vi "Platform Plugin Folder.vi"() -> (2 "Path":path)   [LabVIEW 2020, in "PicoG-Core.lvlib" / "PlatformManager.lvclass"]
uses:
  PlatformManager.lvclass
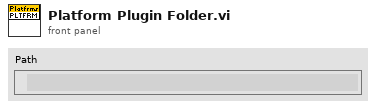
[diagram p1: front panel]
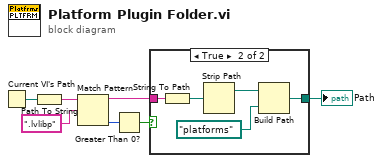
[diagram p0: block diagram]
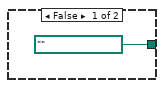
[diagram p2: hidden frame]
diagram:
  n1 = Current VI's Path() -> (path=w7:path)
  n2 = Path To String(path=w7) -> (string=w6:string)
  n3 = Match Pattern(string=w6, regular expression=".lvlibp") -> (before substring=w4:string, offset past match=w2:i32)  [unwired: 1 in, 2 out]
  n4 = Greater Than 0?(x=w2) -> (x > 0?=w1:bool)
  n5 = case shown="True" w1 {
    tunnel: w4 -> [_ w13]
    tunnel: [path "" ("appended path") w9] -> w3
    frame False {
    }
    frame True {
      n6 = String To Path(string=w13) -> (path=w12:path)
      n7 = Strip Path(path=w12) -> (stripped path=w11:path)  [unwired: 1 out]
      n8 = Build Path(base path=w11, name or relative path=path "platforms") -> (appended path=w9:path)
    }
  }
  "Path" <- w3
